vi "Mutate.dotNETConfigFiles.vi"(8 "error in (no error)":errorcluster, 11 "Version Build Information":T1={"VeriStand Version"="2013 SP1", "TestStand Version"="2013", "New VS Assembly Version"="2013.0.0.0", "New TS Assembly Version"="5.1.0.226", "VeriStand Steps Version String"="14.0.5.0", "Project Paths"={"MiscHelperVIs Project Path"="", "RTSequenceVIs Project Path"="", "Set Channels Project Path"="", "TS VS Logger Project Path"="", "VeriStand.exe Install Path"="", "NI_VeristandTypes.ini File Path"="", "Workspace Path"="", "VeristandSteps.csproj File Path"="", "Silent Veristand Project Path"=""}, "New TS Interop Assembly Version"="1.2.3.4", "New TS Utility Assembly Version"="5.6.7.8", "New VS Assembly Version (GAC)"="4.0.2016.0.9.9", "dotNET .config File Paths"={"MiscHelperVIs Project .config File Path"=path "C:/Users/Public/Documents/Git-Source/VeriStand-Custom-Steps-For-TestStand/Source/LabVIEW Code/Misc/MiscHelperVIs.lvproj.config", "RT Sequence VIs Project .config File Path"=path "C:/Users/Public/Documents/Git-Source/VeriStand-Custom-Steps-For-TestStand/Source/LabVIEW Code/RT Sequence/RTSequenceVIs.lvproj.config", "Set Channels Project .config File Path"=path "C:/Users/Public/Documents/Git-Source/VeriStand-Custom-Steps-For-TestStand/Source/LabVIEW Code/Set Channels/Set Channels.lvproj.config", "TS VS Logger Project .config File Path"=path "C:/Users/Public/Documents/Git-Source/VeriStand-Custom-Steps-For-TestStand/Source/LabVIEW Code/TS VS Logger/TS VS Logger.lvproj.config", "Silent Veristand Project .config File Path"=path "C:/Users/Public/Documents/Git-Source/VeriStand-Custom-Steps-For-TestStand/Source/LabVIEW Code/VeriStand Silent Start/SilentVS.lvproj.config"}}) -> (0 "error out":errorcluster, 3 "Version Build Information out":T1={"VeriStand Version"="2013 SP1", "TestStand Version"="2013", "New VS Assembly Version"="2013.0.0.0", "New TS Assembly Version"="5.1.0.226", "VeriStand Steps Version String"="14.0.5.0", "Project Paths"={"MiscHelperVIs Project Path"="", "RTSequenceVIs Project Path"="", "Set Channels Project Path"="", "TS VS Logger Project Path"="", "VeriStand.exe Install Path"="", "NI_VeristandTypes.ini File Path"="", "Workspace Path"="", "VeristandSteps.csproj File Path"="", "Silent Veristand Project Path"=""}, "New TS Interop Assembly Version"="1.2.3.4", "New TS Utility Assembly Version"="5.6.7.8", "New VS Assembly Version (GAC)"="4.0.2016.0.9.9", "dotNET .config File Paths"={"MiscHelperVIs Project .config File Path"=path "C:/Users/Public/Documents/Git-Source/VeriStand-Custom-Steps-For-TestStand/Source/LabVIEW Code/Misc/MiscHelperVIs.lvproj.config", "RT Sequence VIs Project .config File Path"=path "C:/Users/Public/Documents/Git-Source/VeriStand-Custom-Steps-For-TestStand/Source/LabVIEW Code/RT Sequence/RTSequenceVIs.lvproj.config", "Set Channels Project .config File Path"=path "C:/Users/Public/Documents/Git-Source/VeriStand-Custom-Steps-For-TestStand/Source/LabVIEW Code/Set Channels/Set Channels.lvproj.config", "TS VS Logger Project .config File Path"=path "C:/Users/Public/Documents/Git-Source/VeriStand-Custom-Steps-For-TestStand/Source/LabVIEW Code/TS VS Logger/TS VS Logger.lvproj.config", "Silent Veristand Project .config File Path"=path "C:/Users/Public/Documents/Git-Source/VeriStand-Custom-Steps-For-TestStand/Source/LabVIEW Code/VeriStand Silent Start/SilentVS.lvproj.config"}})   [LabVIEW 2014, in "VeriStand Steps Version Mutation.lvlib"]
uses:
  VeriStand Steps Version Mutation.lvlib
  Types/Version Build Information.ctl
  Types/Project Paths Cluster.ctl
  Types/dotNET Config File Paths Cluster.ctl
  <vilib>/xml/Load XML File.vi
  <vilib>/xml/Close Reference(Node).vi
  <vilib>/xml/Close Reference(NNMap).vi
  <vilib>/xml/NI_XML.lvlib
  <resource>/objmgr/DOMUserDefRef.rc
  <vilib>/ni/Simple XML/Simple XML.lvlib
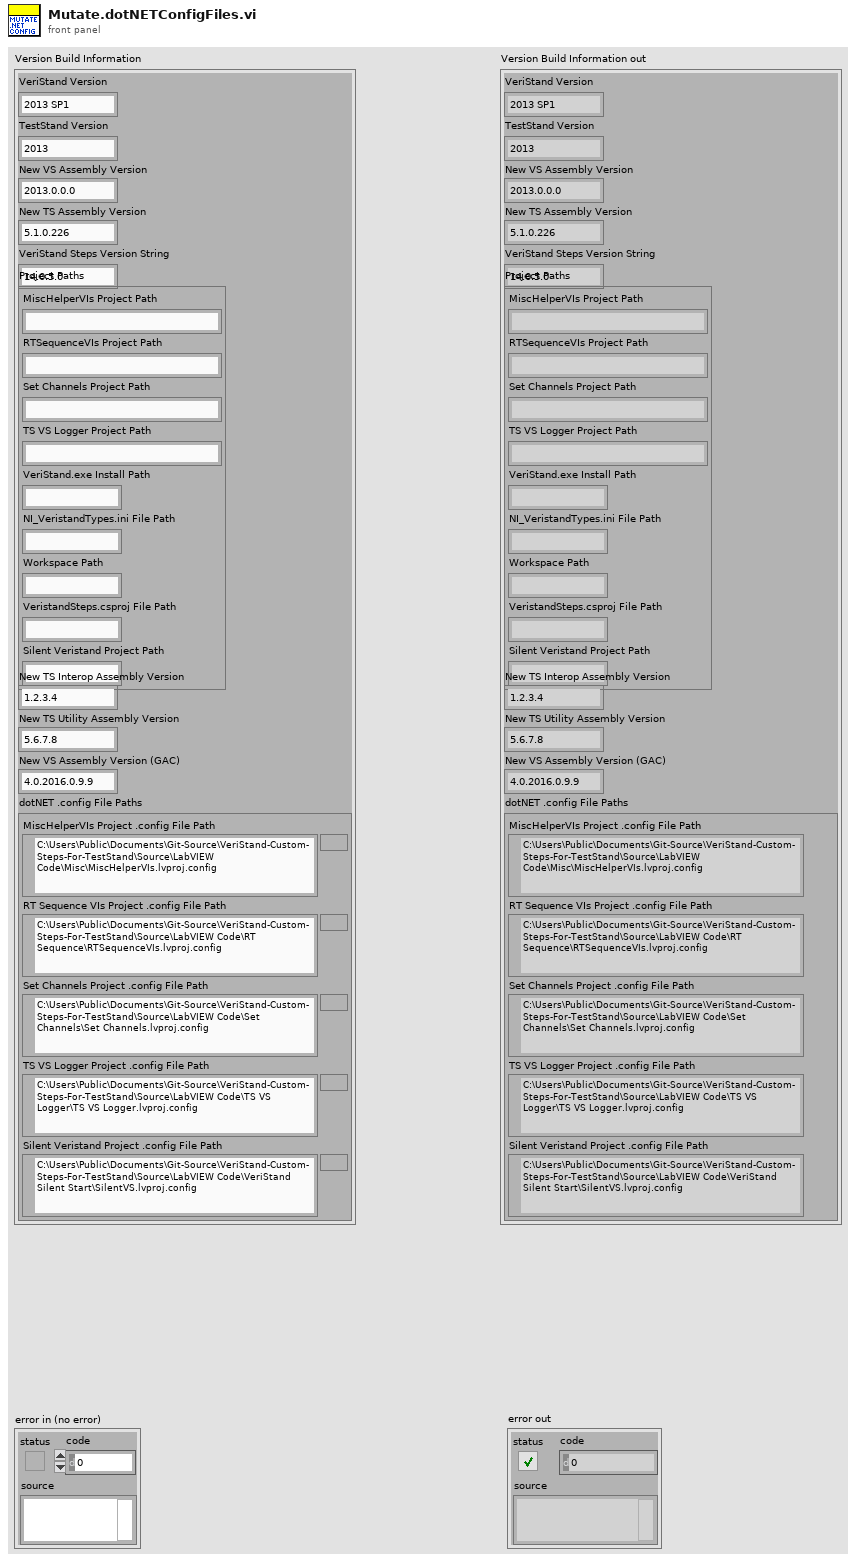
[diagram p1: front panel]
types:
  T1 = typedef "VeriStand Steps Version Mutation.lvlib/Version Build Information.ctl" = cluster{"VeriStand Version":string, "TestStand Version":string, "New VS Assembly Version":string, "New TS Assembly Version":string, "VeriStand Steps Version String":string, "Project Paths":T2, "New TS Interop Assembly Version":string, "New TS Utility Assembly Version":string, "New VS Assembly Version (GAC)":string, "dotNET .config File Paths":T3}
  T2 = typedef "VeriStand Steps Version Mutation.lvlib/Project Paths Cluster.ctl" = cluster{"MiscHelperVIs Project Path":string, "RTSequenceVIs Project Path":string, "Set Channels Project Path":string, "TS VS Logger Project Path":string, "VeriStand.exe Install Path":string, "NI_VeristandTypes.ini File Path":string, "Workspace Path":string, "VeristandSteps.csproj File Path":string, "Silent Veristand Project Path":string}
  T3 = typedef "VeriStand Steps Version Mutation.lvlib/dotNET Config File Paths Cluster.ctl" = cluster{"MiscHelperVIs Project .config File Path":path, "RT Sequence VIs Project .config File Path":path, "Set Channels Project .config File Path":path, "TS VS Logger Project .config File Path":path, "Silent Veristand Project .config File Path":path}
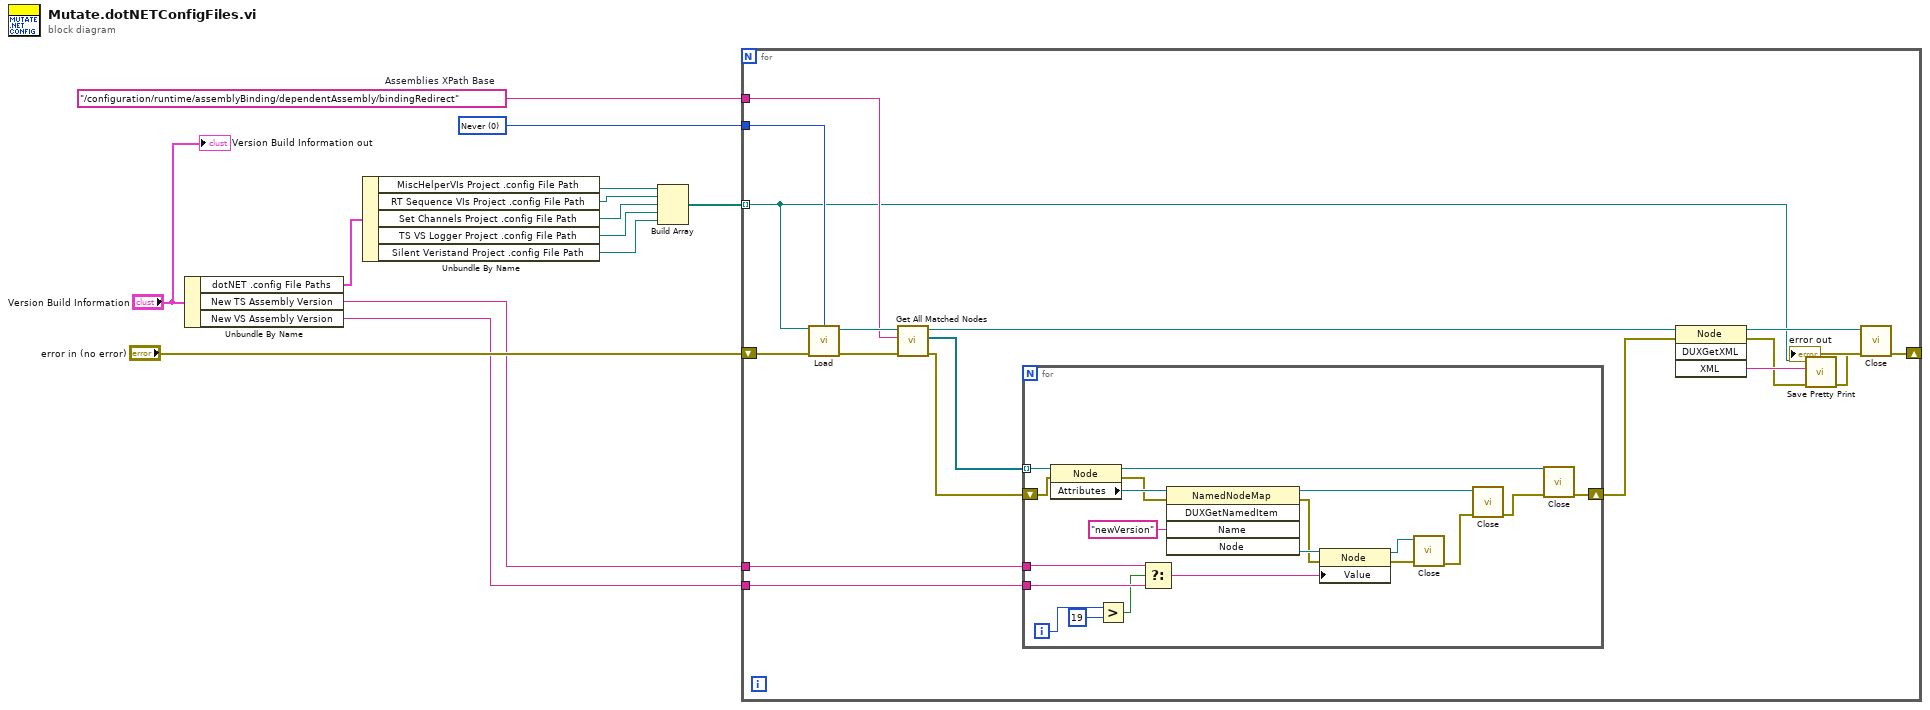
[diagram p0: block diagram]
diagram:
  w13 = "/configuration/runtime/assemblyBinding/dependentAssembly/bindingRedirect"  # Assemblies XPath Base
  w14 = 0 items=["Never", "Always", "Auto"] ("validate on load (Auto)")
  n1 = Unbundle By Name("Version Build Information") -> ("dotNET .config File Paths"=w7:T3, "New TS Assembly Version"=w11:string, "New VS Assembly Version"=w10:string)
  n2 = Unbundle By Name(w7) -> ("MiscHelperVIs Project .config File Path"=w6:path, "RT Sequence VIs Project .config File Path"=w5:path, "Set Channels Project .config File Path"=w4:path, "TS VS Logger Project .config File Path"=w3:path, "Silent Veristand Project .config File Path"=w2:path)
  n3 = Build Array(w6, w5, w4, w3, w2) -> (w1:path[])
  n4 = for {
    tunnel: w14 -> [w31]
    tunnel: w13 -> [w28]
    tunnel: w11 -> [w18]
    tunnel: w10 -> [w17]
    shift-right: [w16] -> w9
    shift-left: "error in (no error)" -> [w19]
    tunnel: w1 -> [w15] mode=indexing
    n5 = call-poly <vilib>:"Load.vi"("path to XML document"=w15, "validate on load (Auto)"=w31, "error in (no error)"=w19) -> ("DOM document out"=w29:refnum<k20>, "error out"=w30:errorcluster)  [unwired: 10 in, 1 out]
    n6 = call <vilib>:"Get All Matched Nodes.vi"("error in (no error)"=w30, "XPath expression"=w28, "node in"=w29) -> ("error out"=w26:errorcluster, "node result array"=w27:refnum<k20>[], "node out"=w24:refnum<k20>)  [unwired: 6 in]
    n7 = for {
      tunnel: w27 -> [w51] mode=indexing
      tunnel: w18 -> [w37]
      shift-right: [w39] -> w25
      shift-left: w26 -> [w48]
      tunnel: w17 -> [w36]
      i -> [w35]
      n8 = property class="Node"(reference=w51, error in=w48) -> (reference out=w41:refnum<k20>, error out=w49:errorcluster, "Attributes"=w50:refnum<k20>)
      n9 = Greater?(x=w35, y=19) -> (0:w33:bool)
      n10 = Select(t=w37, s=w33, f=w36) -> (s? t:f=w32:string)
      n11 = invoke class="NamedNodeMap" method="DUXGetNamedItem"(reference=w50, error in=w49, "Name"="newVersion") -> (reference out=w43:refnum<k20>, error out=w46:errorcluster, "Node"=w47:refnum<k20>)  [unwired: 2 in, 2 out]
      n12 = property class="Node"(reference=w47, error in=w46, "Value"=w32) -> (reference out=w44:refnum<k20>, error out=w45:errorcluster)
      n13 = call-poly <vilib>:"Close.vi"("error in (no error)"=w45, "node"=w44) -> ("error out"=w42:errorcluster)  [unwired: 7 in]
      n14 = call-poly <vilib>:"Close.vi"("error in (no error)"=w42, "named node map"=w43) -> ("error out"=w40:errorcluster)  [unwired: 7 in]
      n15 = call-poly <vilib>:"Close.vi"("error in (no error)"=w40, "node"=w41) -> ("error out"=w39:errorcluster)  [unwired: 7 in]
    }
    n16 = invoke class="Node" method="DUXGetXML"(reference=w24, error in=w25) -> (reference out=w21:refnum<k20>, error out=w22:errorcluster, "XML"=w23:string)  [unwired: 2 in, 1 out]
    n17 = call <vilib>:"Save Pretty Print.vi"("error in (no error)"=w22, "Pretty XML String"=w23, "XML file path"=w15) -> ("error out"=w20:errorcluster)  [unwired: 7 in, 1 out]
    n18 = call-poly <vilib>:"Close.vi"("error in (no error)"=w20, "node"=w21) -> ("error out"=w16:errorcluster)  [unwired: 7 in]
  }
  "error out" <- w9
  "Version Build Information out" <- "Version Build Information"
